vi "初始化.vi"(11 "地图编号":enum16{"无迷宫", "方盒", "铁道", "工厂"}(ring)) -> (0 "行列数":i32, 1 "方向":enum16{"左", "右", "上", "下"}(ring), 2 "蛇":cluster{"x":dbl, "y":dbl}[](array[cluster]), 3 "地图":u32[][](array[colorbox]), 4 "初始位置":cluster{"x":dbl, "y":dbl}={"x"=1.0, "y"=10.0})   [LabVIEW 2012]
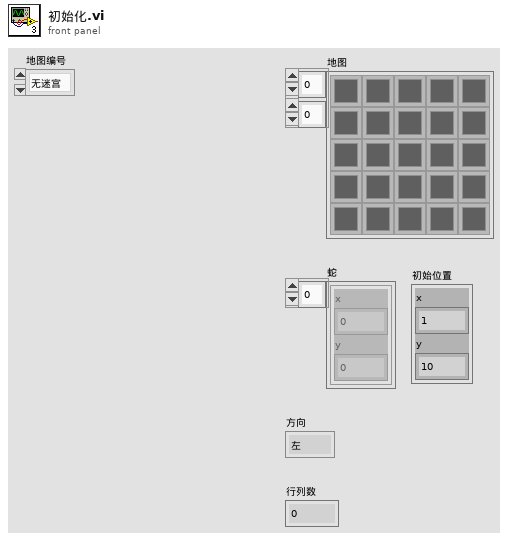
[diagram p1: front panel]
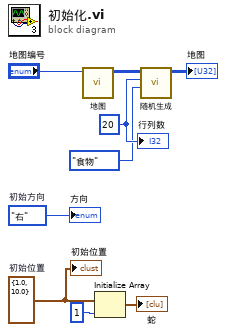
[diagram p0: block diagram]
diagram:
  w3 = enum16{"左", "右", "上", "下"}."右"  # 初始方向
  w6 = cluster{"x":dbl, "y":dbl} {"x"=1.0, "y"=10.0}  # 初始位置
  w2 = 20 ("行列数")
  n1 = call "地图.vi"("地图编号"="地图编号") -> ("地图"=w8:u32[][])  [unwired: 10 in]
  n2 = Initialize Array(w6, 1 ("维数大小")) -> (→"蛇":cluster{"x":dbl, "y":dbl}[])
  n3 = call "随机生成.vi"("类型"=enum16{"空白", "蛇", "食物", "墙", "传送门"}."食物", "上限"=w2, "地图"=w8) -> ("地图 2"=→"地图":u32[][])  [unwired: 8 in]
  "行列数" <- w2
  "方向" <- w3
  "初始位置" <- w6
